vi "Method.vi"(8 "error in (no error)":errorcluster, 11 "Abstract Class in":refnum<class "Abstract Class.lvclass">) -> (0 "error out":errorcluster, 3 "Abstract Class out":refnum<class "Abstract Class.lvclass">)   [LabVIEW 2021, in "Abstract Class.lvclass"]
uses:
  Abstract Class.lvclass
  Abstract Class.lvclass/Abstract Class.ctl
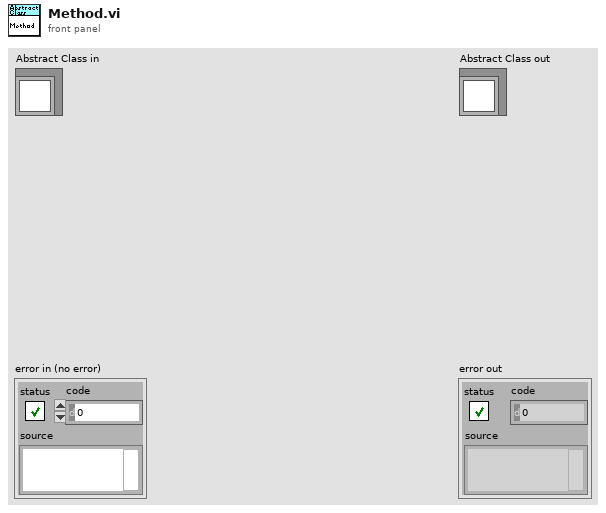
[diagram p1: front panel]
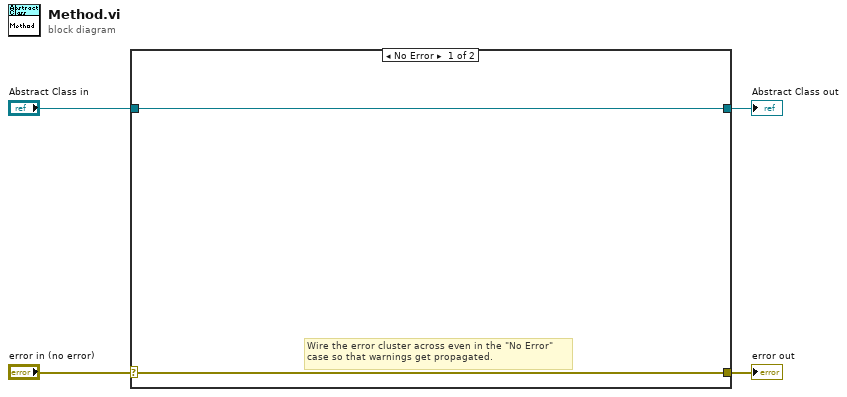
[diagram p0: block diagram]
diagram:
  n1 = case shown="No Error" "error in (no error)" {
    selector: "error in (no error)" -> [w5 w8]
    tunnel: [w5 w8] -> w3
    tunnel: [w6 w7] -> w1
    tunnel: "Abstract Class in" -> [w6 w7]
    frame No Error {
      # "Wire the error cluster across even in the \"No Error\"\ncase so that warnings get propagated."
    }
    frame Error {
    }
  }
  "error out" <- w3
  "Abstract Class out" <- w1
